vi "Do Set Value.vi"(8 "error in (no error)":errorcluster, 10 "set_value Argument":T2, 11 "Data Cluster in":T1) -> (0 "error out":errorcluster, 3 "Data Cluster out":T1)   [LabVIEW 2025, in "Scripting Server.lvlib"]
uses:
  Scripting Server.lvlib
  Module Data--cluster.ctl
  set_value (Reply Payload)--cluster.ctl
  set_value Argument--cluster.ctl
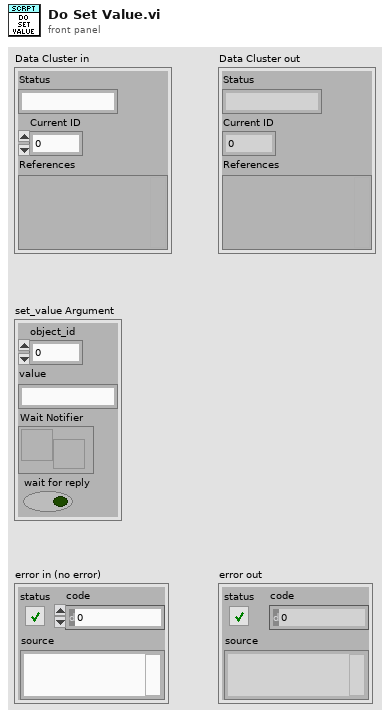
[diagram p1: front panel]
types:
  T1 = typedef "Scripting Server.lvlib/Module Data--cluster.ctl" = cluster{"Status":string, "Current ID":i32, "References":variant}
  T2 = typedef "Scripting Server.lvlib/set_value Argument--cluster.ctl" = cluster{"object_id":i32, "value":string, "Wait Notifier":refnum<notifier>, "wait for reply":bool}
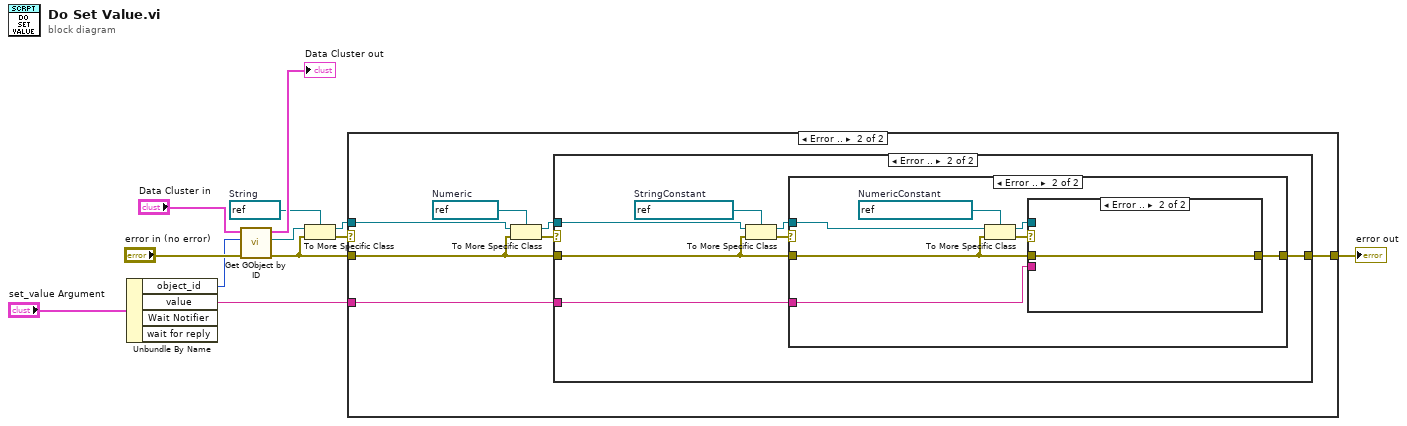
[diagram p0: block diagram]
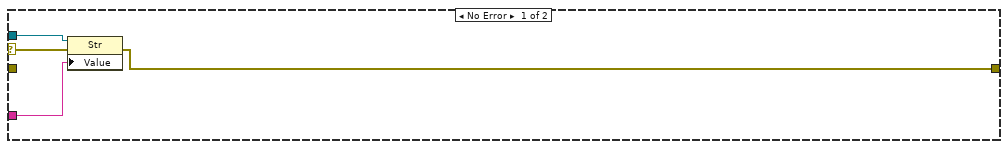
[diagram p2: hidden frame]
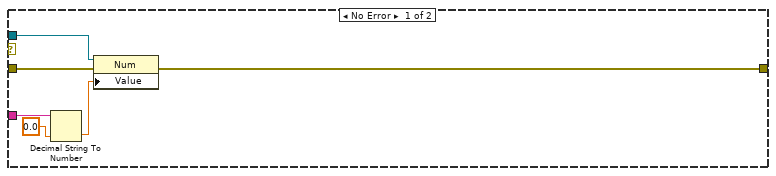
[diagram p3: hidden frame]
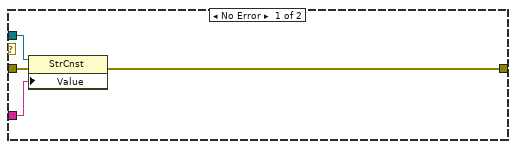
[diagram p4: hidden frame]
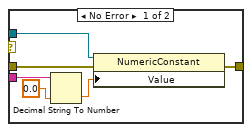
[diagram p5: hidden frame]
diagram:
  w6 = refnum<vi> refnum  # String
  n1 = Unbundle By Name("set_value Argument") -> ("object_id"=w8:i32, "value"=w1:string)  [unwired: 2 out]
  n2 = call "Get GObject by ID.vi"("error in (no error)"="error in (no error)", "ID"=w8, "Data Cluster in"="Data Cluster in") -> ("error out"=w2:errorcluster, "gobject"=w7:refnum<vi>, "Data Cluster out"=→"Data Cluster out":T1)  [unwired: 6 in]
  n3 = To More Specific Class(target class=w6, reference=w7, error in=w2) -> (specific class reference=w3:refnum<vi>, error out=w4:errorcluster)
  n4 = case shown="Error .." w4 {
    selector: w4 -> [w15 _]
    tunnel: [w16 w21] -> w5
    tunnel: w3 -> [w14 w23]
    tunnel: w2 -> [_ w18]
    tunnel: w1 -> [w13 w17]
    frame No Error {
      n5 = property class="Str"(reference=w14, error in=w15, "Value"=w13) -> (error out=w16:errorcluster)  [unwired: 1 out]
    }
    frame Error {
      w22 = refnum<vi> refnum  # Numeric
      n6 = To More Specific Class(target class=w22, reference=w23, error in=w18) -> (specific class reference=w20:refnum<vi>, error out=w19:errorcluster)
      n7 = case shown="Error .." w19 {
        tunnel: [w29 w33] -> w21
        tunnel: w20 -> [w28 w35]
        tunnel: w18 -> [w27 w34]
        tunnel: w17 -> [w26 w30]
        frame No Error {
          n8 = Decimal String To Number(string=w26, default (0L)=0.0) -> (number=w25:dbl)  [unwired: 1 in, 1 out]
          n9 = property class="Num"(reference=w28, error in=w27, "Value"=w25) -> (error out=w29:errorcluster)  [unwired: 1 out]
        }
        frame Error {
          w36 = refnum<vi> refnum  # StringConstant
          n10 = To More Specific Class(target class=w36, reference=w35, error in=w34) -> (specific class reference=w32:refnum<vi>, error out=w31:errorcluster)
          n11 = case shown="Error .." w31 {
            tunnel: w34 -> [w40 w46]
            tunnel: [w39 w45] -> w33
            tunnel: w32 -> [w38 w41]
            tunnel: w30 -> [w37 w43]
            frame No Error {
              n12 = property class="StrCnst"(reference=w38, error in=w40, "Value"=w37) -> (error out=w39:errorcluster)  [unwired: 1 out]
            }
            frame Error {
              w47 = refnum<vi> refnum  # NumericConstant
              n13 = To More Specific Class(target class=w47, reference=w41, error in=w46) -> (specific class reference=w44:refnum<vi>, error out=w42:errorcluster)
              n14 = case shown="Error .." w42 {
                tunnel: w46 -> [w53 w54]
                tunnel: [w52 w54] -> w45
                tunnel: w44 -> [w51 _]
                tunnel: w43 -> [w49 _]
                frame No Error {
                  n15 = Decimal String To Number(string=w49, default (0L)=0.0) -> (number=w48:dbl)  [unwired: 1 in, 1 out]
                  n16 = property class="NumericConstant"(reference=w51, error in=w53, "Value"=w48) -> (error out=w52:errorcluster)  [unwired: 1 out]
                }
                frame Error {
                }
              }
            }
          }
        }
      }
    }
  }
  "error out" <- w5
